vi "Target2.vi"() -> ()   [LabVIEW 2025]
uses:
  <vilib>/Platform/TimedLoop/XDataNode/timing_clust.ctl
  <vilib>/Platform/TimedLoop/XDataNode/nitl_modes.ctl
  <vilib>/Platform/TimedLoop/XDataNode/wakeup.ctl
  <vilib>/eio/utilities/niEioResolveVilibRelativePath.vi
  <vilib>/rvi/interface/RandomDataEmulation/niFpgaRandomDataHandleErrors.vi
  <vilib>/rvi/Emulation/niFpgaSctlEmulationGetInTimedLoop.vi
  <vilib>/rvi/Emulation/niFpgaEmulationReportErrorSimple.vi
  <vilib>/rvi/Emulation/niFpgaGetClockAttributes.vi
  <vilib>/rvi/Emulation/niFpgaCriticalErrorInLSC.vi
  <vilib>/rvi/interface/RandomDataEmulation/nirviRandomDataMultiElementFPGAFIFO.vi
  <instcachedir>/0/nirviRandomDataMultiElementFPGAFIFO_BE2FF10D3D6E420AB0291A02835C249E.lvgen/nirviRandomDataMultiElementFPGAFIFO_BE2FF10D3D6E420AB0291A02835C249E_001.vi
  <vilib>/rvi/DataTransferAndStorage/Container/XNode/niFpgaContainer.xnode
  <vilib>/rvi/interface/RandomDataEmulation/nirviRandomDataFpgaReadWriteTemplate.vi
  <vilib>/platform/TimedLoop/XDataNode/XDataNode.xnode
  <vilib>/rvi/interface/RandomDataEmulation/nirviRandomDataFpgaMultiElementTemplate.vi
  <vilib>/Platform/TimedLoop/XDataNode/XDNodeRunTimeDep.lvlib
panel:
  out "Array 2":fxp<+/-,32,16>[](array[numeric])
  out "Array 1":fxp<+/-,32,16>[](array[numeric])
  out "appended array":fxp<+/-,32,16>[](array[numeric])
  out "appended array 2":fxp<+/-,32,16>[](array[numeric])
  out "element":fxp<+/-,32,16>
  out "element 2":fxp<+/-,32,16>
  out "element 3":fxp<+/-,32,16>
  out "element 4":fxp<+/-,32,16>
  out "Array 1.2":fxp<+/-,32,16>[](array[numeric])
  out "Array 2.1":fxp<+/-,32,16>[](array[numeric])
  out "cr":fxp<+/-,32,16>[](array[numeric])
  out "Numeric":i32
  out "Case Number":i16
  out "interleaved array":fxp<+/-,32,16>[](array[numeric])
  out "interleaved array 2":fxp<+/-,32,16>[](array[numeric])
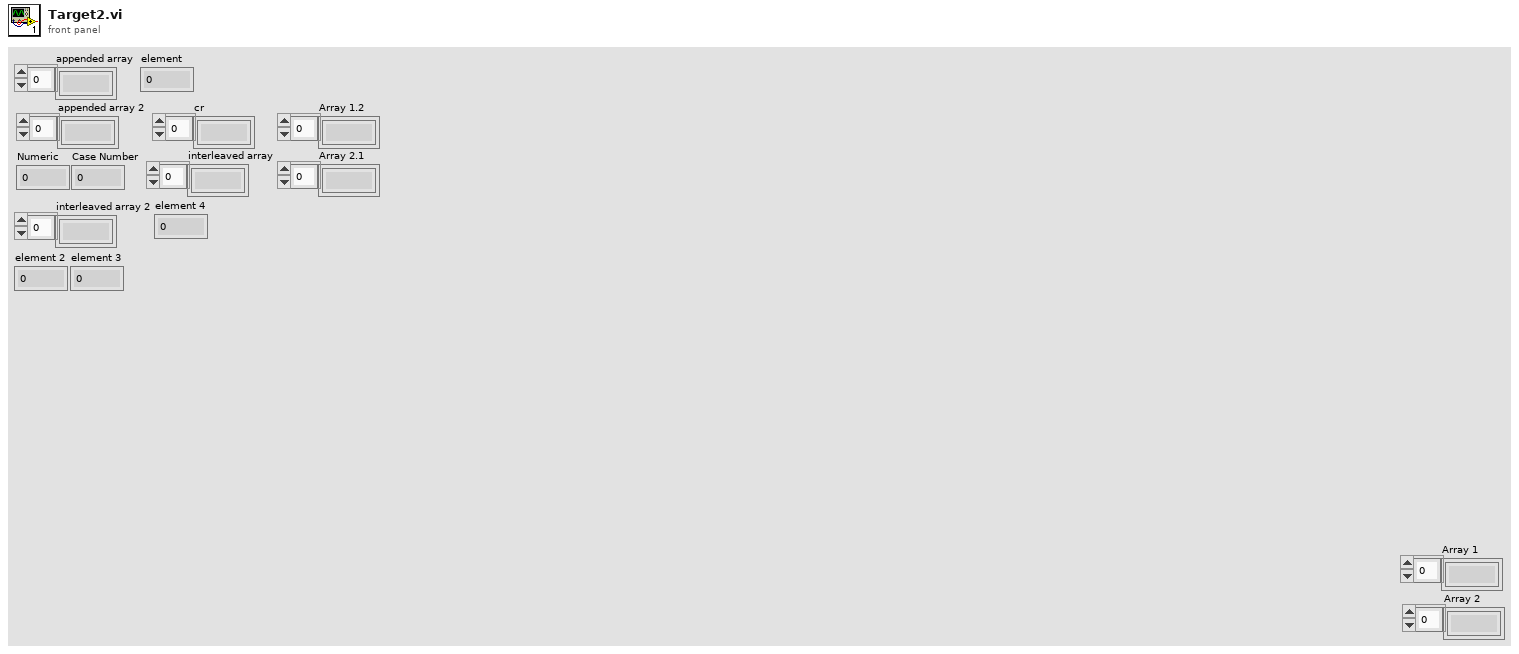
[diagram p1: front panel]
types:
  T1 = typedef "XDNodeRunTimeDep.lvlib/timing_clust.ctl" = cluster{"Expected End [f-1]":u64, "Actual End [f-1]":u64, "Finished Late? [f-1]":bool, "Expected End [i-1]":u64, "Actual End [i-1]":u64, "Finished Late? [i-1]":bool, "Expected Start [i]":u64, "Actual Start [i]":u64, "Expected Start [f]":u64, "Actual Start [f]":u64, "Source Name":string, "Structure Name":string, "Period":i64, "Deadline":i64, "Offset":i64, "Start":i64, "Priority":i32, "Timeout":i32, "Mode":T2, "Wakeup Reason":T3, "Error":errorcluster, "Source Type":string, "Secondary Source Type":string, "Global End Time":u64, "Global Start Time":u64, "Frame Duration":u64, "Iteration Duration":u64, "Assigned CPU":i32, "I/O Scan Engine Mode":u32}
  T2 = typedef "XDNodeRunTimeDep.lvlib/nitl_modes.ctl" = enum32{"No Change", "Process missed periods, maintain original phase", "Discard missed periods, maintain original phase", "Process missed periods, ignore original phase", "Discard missed periods, ignore original phase"}
  T3 = typedef "XDNodeRunTimeDep.lvlib/wakeup.ctl" = enum32{"Normal", "Aborted", "Asynchronous wakeup", "Timing source error", "Timed loop error", "Timeout"}
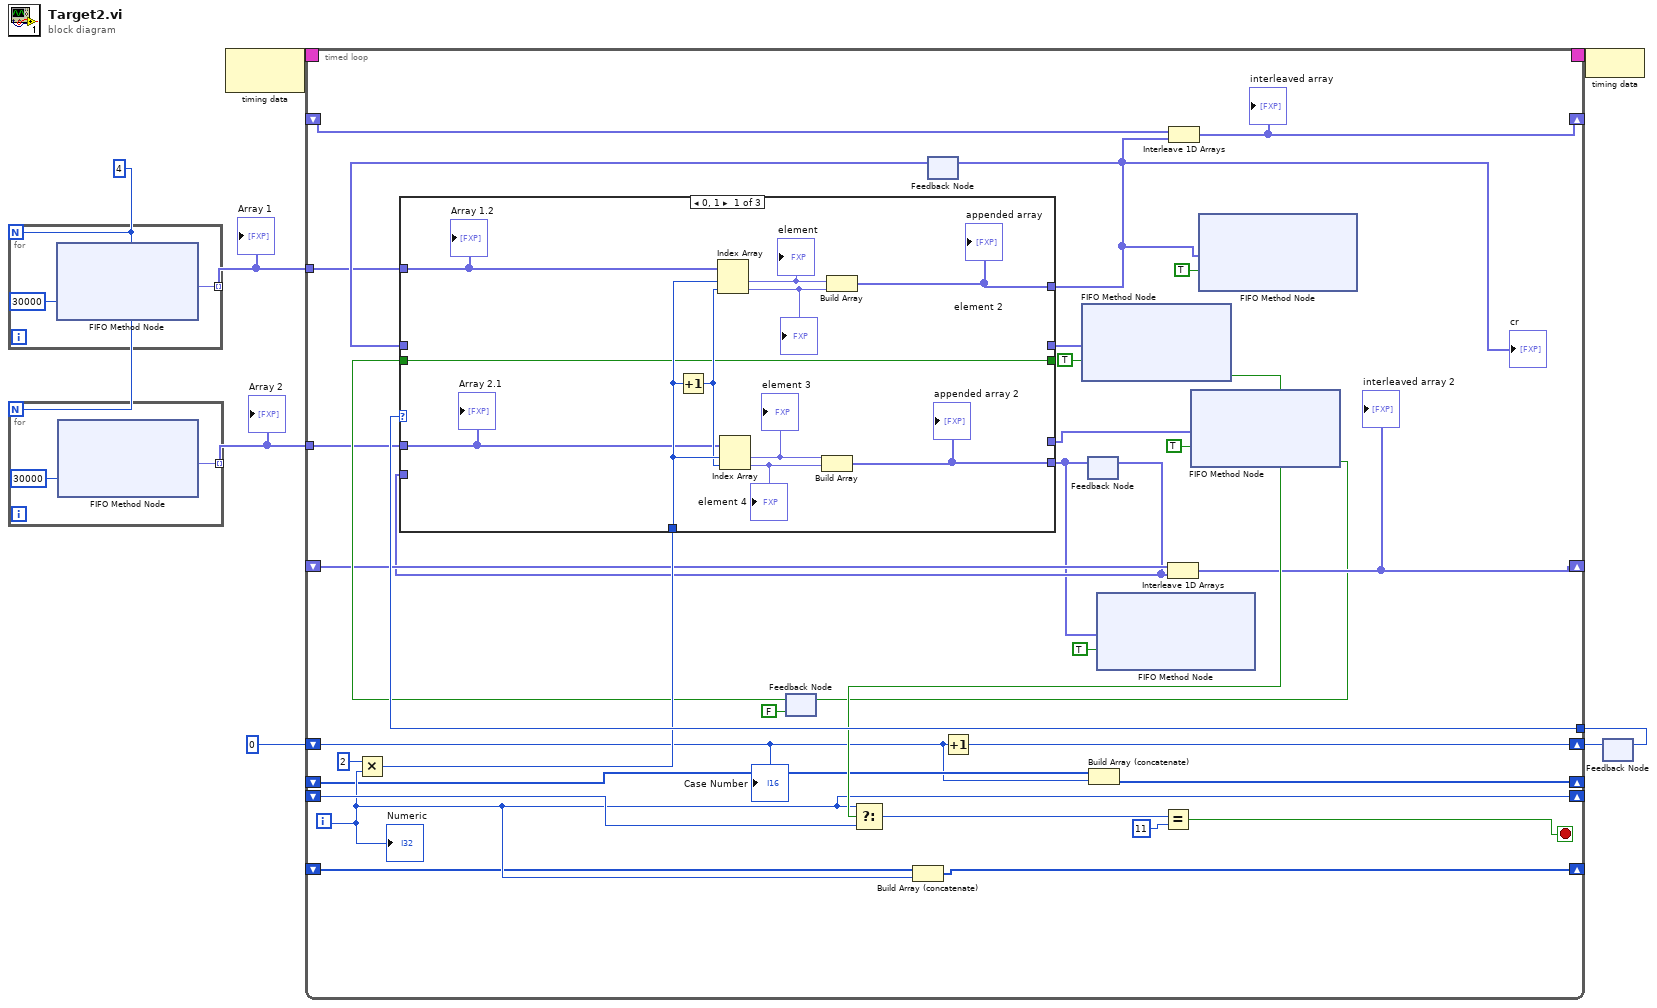
[diagram p0: block diagram]
diagram:
  w3 = 4
  n1 = for {
    N: w3 -> [_]
    tunnel: [w10] -> w2 mode=indexing
    n2 = xnode ("FIFO Method Node")("Timeout"=30000) -> ("Element"=w10:fxp<+/-,32,16>)  [unwired: 1 in, 2 out]
  }
  "Array 1" <- w2
  n3 = for {
    N: w3 -> [_]
    tunnel: [w12] -> w1 mode=indexing
    n4 = xnode ("FIFO Method Node")("Timeout"=30000) -> ("Element"=w12:fxp<+/-,32,16>)  [unwired: 1 in, 2 out]
  }
  "Array 2" <- w1
  n5 = node-c288() -> (w8:T1)  [unwired: 1 in]
  n6 = feedback #1() -> (w4:i16)  [unwired: 1 in]
  n7 = timed-loop {
    timing: w8 -> [_]
    timing-out: [_] -> w7
    shift-right: [w46] -> w5
    shift-left: i16 0 -> [w22]
    tunnel: w4 -> [w45]
    shift-right: [w27] -> _
    shift-left: _ -> [w41]
    tunnel: w2 -> [w35]
    tunnel: w1 -> [w34]
    shift-right: [w29] -> _
    shift-left: _ -> [w30]
    shift-right: [w28] -> _
    shift-left: _ -> [w31]
    shift-right: [w25] -> _
    shift-left: _ -> [w26]
    shift-right: [w23] -> _
    shift-left: _ -> [w24]
    i -> [w27]
    stop <- w38 stop-if-true
    n8 = Multiply(x=2, y=w27) -> (x*y=w43:i32)
    n9 = feedback #2(FALSE ("output valid")) -> (w37:bool)
    n10 = Build Array (concatenate)(w26, w27) -> (w25:i32[])
    n11 = feedback #3() -> (w42:fxp<+/-,32,16>[])  [unwired: 1 in]
    n12 = Increment(x=w22) -> (x+1=w46:i16)
    n13 = feedback #4() -> (w21:fxp<+/-,32,16>[])  [unwired: 1 in]
    n14 = case shown="0, 1" w45 {
      tunnel: [w53 _ _] -> w16
      tunnel: [w52 _ _] -> w13
      tunnel: w43 -> [w51 _ _]
      tunnel: w42 -> [_ _ w61]
      tunnel: w37 -> [w47 w58 w60]
      tunnel: w35 -> [w49 _ _]
      tunnel: w34 -> [w48 _ _]
      tunnel: [_ _ w61] -> w32
      tunnel: [w47 w58 w60] -> _
      tunnel: w21 -> [_ _ w59]
      tunnel: [_ _ w59] -> w20
      frame 0, 1 {
        n15 = Increment(x=w51) -> (x+1=w50:i32)
        n16 = Index Array(array=w49, index #1=w51, index #2=w50) -> (element #1=w55:fxp<+/-,32,16>, element #2=w54:fxp<+/-,32,16>)
        "element" <- w55
        "element 2" <- w54
        n17 = Index Array(array=w48, index #1=w51, index #2=w50) -> (element #1=w57:fxp<+/-,32,16>, element #2=w56:fxp<+/-,32,16>)
        "element 3" <- w57
        "element 4" <- w56
        n18 = Build Array(w57, w56) -> (w52:fxp<+/-,32,16>[])
        "appended array 2" <- w52
        n19 = Build Array(w55, w54) -> (w53:fxp<+/-,32,16>[])
        "appended array" <- w53
        "Array 1.2" <- w49
        "Array 2.1" <- w48
      }
      frame 3, Default {
      }
      frame 10, 11 {
      }
    }
    "cr" <- w16
    n20 = feedback-in #3(w16) -> ()
    n21 = xnode ("FIFO Method Node")("Element"=w32, "Input Valid"=TRUE) -> ("Ready for Input"=w33:bool)  [unwired: 1 in, 1 out]
    n22 = Select(t=w27, s=w33, f=w41) -> (s? t:f=w40:i32)
    n23 = feedback-in #4(w13) -> ()
    n24 = Build Array (concatenate)(w24, w22) -> (w23:i16[])
    n25 = xnode ("FIFO Method Node")("Element"=w13, "Input Valid"=TRUE) -> ()  [unwired: 1 in, 2 out]
    n26 = Equal?(x=w40, y=11) -> (x = y?=w38:bool)
    n27 = Interleave 1D Arrays(w31, w21) -> (w28:fxp<+/-,32,16>[])
    "interleaved array 2" <- w28
    n28 = Interleave 1D Arrays(w30, w16) -> (w29:fxp<+/-,32,16>[])
    "interleaved array" <- w29
    n29 = xnode ("FIFO Method Node")("Element"=w20, "Input Valid"=TRUE) -> ("Ready for Input"=w19:bool)  [unwired: 1 in, 1 out]
    n30 = feedback-in #2(w19) -> ()
    n31 = xnode ("FIFO Method Node")("Element"=w16, "Input Valid"=TRUE) -> ()  [unwired: 1 in, 2 out]
    "Numeric" <- w27
    "Case Number" <- w22
  }
  n32 = node-c288(w7) -> ()
  n33 = feedback-in #1(w5) -> ()
